vi "Compile & Log Data.vi"(8 "error in (no error)":errorcluster, 11 "SV B-M (Host) in":refnum<class "SV B-M (Host).lvclass">) -> (0 "error out":errorcluster, 3 "SV B-M (Host) out":refnum<class "SV B-M (Host).lvclass">)   [LabVIEW 2015, in "SV B-M (Host).lvclass"]
uses:
  SV B-M (Host).lvclass
  SV B-M (Host).lvclass/SV B-M (Host).ctl
  Listbox - In Progress.vi
  Listbox - Complete.vi
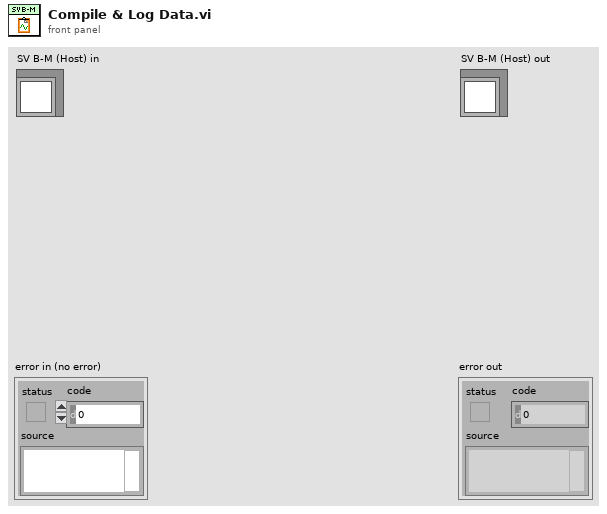
[diagram p1: front panel]
types:
  T1 = enum16{"open", "open or create", "create or replace", "create", "open (read-only)"}
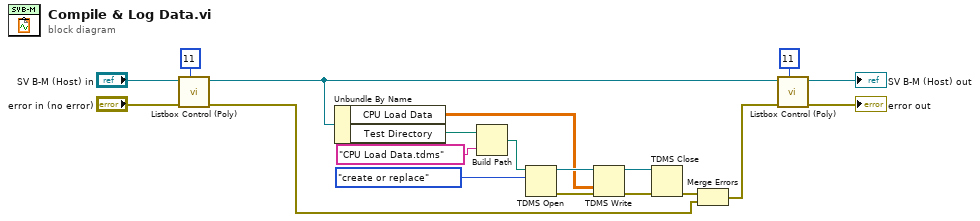
[diagram p0: block diagram]
diagram:
  n1 = call-poly "Listbox Control (Poly).vi"("Row to Update"=11, "error in (no error)"="error in (no error)", "SV B-M In"="SV B-M (Host) in") -> ("error out"=w2:errorcluster, "SV B-M Out"=w19:refnum<class "SV B-M (Host).lvclass">)  [unwired: 7 in]
  n2 = Unbundle By Name(w19) -> ("CPU Load Data"=w6:dbl[][], "Test Directory"=w12:path)
  n3 = Build Path(base path=w12, name or relative path="CPU Load Data.tdms") -> (appended path=w9:path)
  n4 = TDMS Open(10:T1."create or replace" ("operation (0:open)"), 11:w9) -> (0:w7:errorcluster, 3:w8:refnum<k34>)  [unwired: 5 in]
  n5 = TDMS Write(0:w8, 9:w6, 11:w7) -> (4:w5:refnum<k34>, 15:w4:errorcluster)  [unwired: 3 in, 2 out]
  n6 = TDMS Close(8:w4, 11:w5) -> (0:w3:errorcluster)  [unwired: 1 out]
  n7 = Merge Errors(w3, w2) -> (w1:errorcluster)
  n8 = call-poly "Listbox Control (Poly).vi"("Row to Update"=11, "error in (no error)"=w1, "SV B-M In"=w19) -> ("error out"=→"error out":errorcluster, "SV B-M Out"=→"SV B-M (Host) out":refnum<class "SV B-M (Host).lvclass">)  [unwired: 7 in]
